vi "sv_Filter Even-Angle Signal for Specific Notch.vi"(0 "even-angle signals":cluster{"r0":dbl, "dr":dbl, "Y":dbl[]}[](array[cluster]), 2 "reset?":bool, 7 "even-angle position info":T1, 9 "notch harmonic":dbl=1.0 format="%0.2f", 11 "error in (no error)":errorcluster, 12 "bandwidth [order]":dbl=1.0 format="%0.2f", 13 "zero delay? (F)":bool) -> (4 "even-angle signals out":cluster{"r0":dbl, "dr":dbl, "Y":dbl[]}[](array[cluster]), 8 "even-angle position info out":T1, 10 "delay [samples]":i32, 15 "error out":errorcluster)   [LabVIEW 2017, in "SoundVib_ContSweptSine.lvlib"]
uses:
  <vilib>/addons/Sound and Vibration/svt_Continuous Swept Sine/SoundVib_ContSweptSine.lvlib
  <vilib>/addons/Sound and Vibration/Order Analysis/Misc/OAT Position Info.ctl
  <vilib>/Analysis/3filter.llb/FIR Filter with I.C. (DBL).vi
  <vilib>/Analysis/NI_AALBase.lvlib
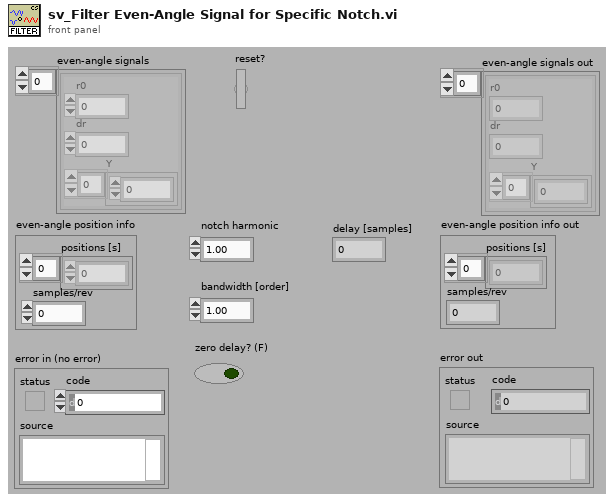
[diagram p1: front panel]
types:
  T1 = typedef "OAT Position Info.ctl" = cluster{"positions [s]":dbl[], "samples/rev":dbl}
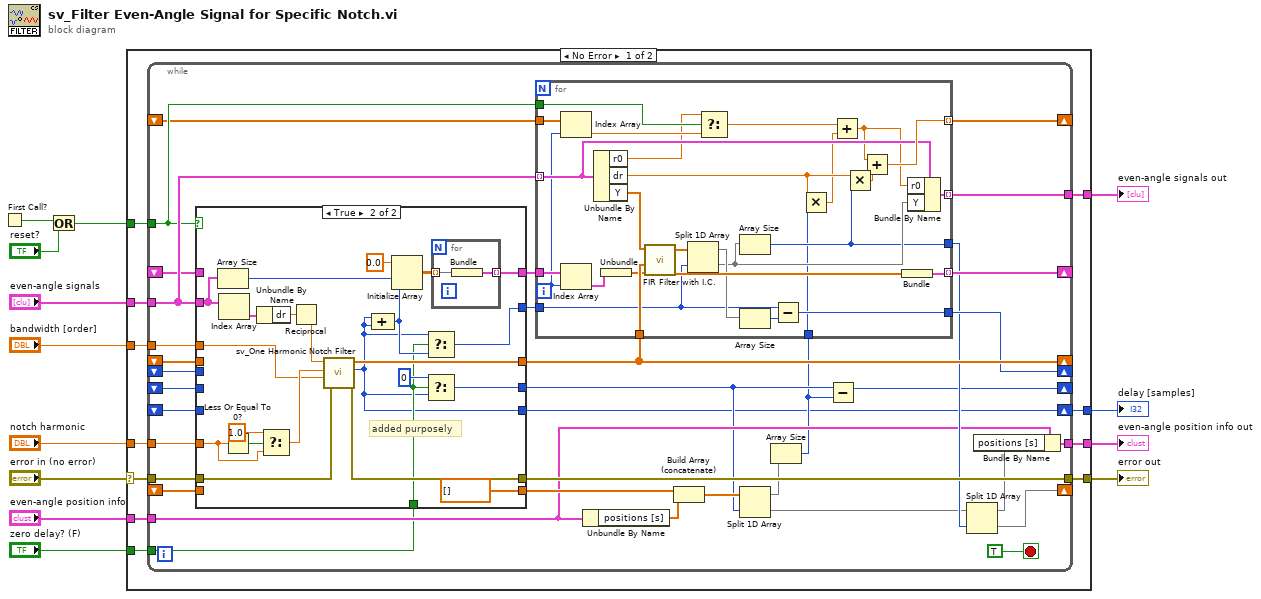
[diagram p0: block diagram]
diagram:
  n1 = First Call?() -> (First Call?: T/F=w13:bool)
  n2 = Or(x=w13, y="reset?") -> (x .or. y?=w11:bool)
  n3 = case shown="No Error" "error in (no error)" {
    selector: "error in (no error)" -> [w20 w123]
    tunnel: w11 -> [w24 _]
    tunnel: "even-angle signals" -> [w23 w122]
    tunnel: "notch harmonic" -> [w22 _]
    tunnel: [w21 w122] -> w8
    tunnel: [w19 w123] -> w6
    tunnel: "even-angle position info" -> [w18 w121]
    tunnel: [w17 w121] -> w4
    tunnel: "zero delay? (F)" -> [w16 _]
    tunnel: [w15 _] -> w2
    tunnel: "bandwidth [order]" -> [w14 _]
    frame No Error {
      n4 = while {
        tunnel: w24 -> [w52]
        tunnel: w23 -> [w55]
        tunnel: w22 -> [w59]
        shift-right: [w54] -> _
        shift-left: _ -> [w58]
        shift-right: [w53] -> _
        shift-left: _ -> [w48]
        shift-right: [w56] -> _
        shift-left: _ -> [w47]
        shift-right: [w51] -> _
        shift-left: _ -> [w50]
        tunnel: [w49] -> w21
        tunnel: w20 -> [w46]
        tunnel: [w45] -> w19
        tunnel: w18 -> [w37]
        shift-right: [w42] -> _
        shift-left: _ -> [w41]
        tunnel: [w36] -> w17
        shift-right: [w32] -> _
        shift-left: _ -> [w31]
        tunnel: w16 -> [w30]
        shift-right: [w25] -> w15
        shift-left: _ -> [w27]
        tunnel: w14 -> [w26]
        stop <- TRUE stop-if-true
        n5 = case shown="True" w52 {
          tunnel: w55 -> [_ w114]
          tunnel: w59 -> [_ w107]
          tunnel: [w95 w116] -> w54
          tunnel: w58 -> [w95 _]
          tunnel: [w94 w111] -> w57
          tunnel: w48 -> [w90 _]
          tunnel: w47 -> [w94 _]
          tunnel: w46 -> [w93 w110]
          tunnel: [w93 w109] -> w45
          tunnel: w41 -> [w92 _]
          tunnel: [w92 dbl[] []] -> w39
          tunnel: [w91 w99] -> w35
          tunnel: w31 -> [w91 _]
          tunnel: w30 -> [_ w100]
          tunnel: [w90 w102] -> w29
          tunnel: w27 -> [w89 _]
          tunnel: w26 -> [_ w97]
          tunnel: [w89 w96] -> w25
          frame False {
          }
          frame True {
            # "added purposely"
            n6 = Array Size(array=w114) -> (size(s)=w113:i32)
            n7 = Index Array(array=w114) -> (element=w118:cluster{"r0":dbl, "dr":dbl, "Y":dbl[]})  [unwired: 1 in]
            n8 = Less Or Equal To 0?(x=w107) -> (x <= 0?=w108:bool)
            n9 = Unbundle By Name(w118) -> ("dr"=w98:dbl)
            n10 = Select(t=1.0, s=w108, f=w107) -> (s? t:f=w105:dbl)
            n11 = Reciprocal(x=w98) -> (1/x=w117:dbl)
            n12 = call <vilib>:"sv_One Harmonic Notch Filter.vi"("error in (no error)"=w110, "bandwidth [order]"=w97, "specific harmonic"=w105, "fs"=w117) -> ("error out"=w109:errorcluster, "delay [samples]"=w96:i32, "FIR filter"=w116:dbl[])  [unwired: 5 in]
            n13 = Compound Arithmetic op=ADD(w96, w96) -> (w103:i32)
            n14 = Initialize Array(0.0 ("element"), w113, w103) -> (w112:dbl[][])
            n15 = Select(t=w96, s=w100, f=w103) -> (s? t:f=w102:i32)
            n16 = Select(t=0, s=w100, f=w96) -> (s? t:f=w99:i32)
            n17 = for {
              tunnel: w112 -> [w120] mode=indexing
              tunnel: [w119] -> w111 mode=indexing
              n18 = Bundle(w120) -> (w119:cluster{dbl[]})  [unwired: 1 in]
            }
          }
        }
        n19 = Unbundle By Name(w37) -> ("positions [s]"=w44:dbl[])
        n20 = Build Array (concatenate)(w39, w44) -> (w40:dbl[])
        n21 = Split 1D Array(array=w40, index=w35) -> (first subarray=w33:dbl[], second subarray=w34:dbl[])
        n22 = Array Size(array=w33) -> (size(s)=w28:i32)
        n23 = for {
          tunnel: w57 -> [w88]
          tunnel: [w74] -> w56 mode=indexing
          tunnel: w55 -> [w79] mode=indexing
          tunnel: w54 -> [w85]
          tunnel: [w83] -> w53
          tunnel: w52 -> [w77]
          tunnel: [w80] -> w51 mode=indexing
          tunnel: w50 -> [w76]
          tunnel: [w75] -> w49 mode=indexing
          tunnel: [w69] -> w43
          tunnel: w29 -> [w68]
          tunnel: w28 -> [w66]
          i -> [w70]
          n24 = Index Array(array=w76, index=w70) -> (element=w72:dbl)
          n25 = Index Array(array=w88, index=w70) -> (element=w71:cluster{"Final X Conditions":dbl[]})
          n26 = Unbundle By Name(w79) -> ("r0"=w63:dbl, "dr"=w65:dbl, "Y"=w86:dbl[])
          n27 = Unbundle(w71) -> ("Final X Conditions"=w73:dbl[])
          n28 = call-poly <vilib>:"FIR Filter with I.C..vi"("Initial X Conditions"=w73, "FIR Coefficients"=w85, "X"=w86) -> ("Final X Conditions"=w87:dbl[], "Filtered X"=w84:dbl[])  [unwired: 5 in, 1 out]
          n29 = Split 1D Array(array=w84, index=w68) -> (first subarray=w82:dbl[], second subarray=w78:dbl[])
          n30 = Select(t=w63, s=w77, f=w72) -> (s? t:f=w62:dbl)
          n31 = Array Size(array=w78) -> (size(s)=w69:i32)
          n32 = Array Size(array=w82) -> (size(s)=w67:i32)
          n33 = Subtract(x=w68, y=w67) -> (x-y=w83:i32)
          n34 = Multiply(x=w65, y=w66) -> (x*y=w64:dbl)
          n35 = Add(x=w62, y=w64) -> (x+y=w61:dbl)
          n36 = Multiply(x=w65, y=w69) -> (x*y=w81:dbl)
          n37 = Add(x=w61, y=w81) -> (x+y=w80:dbl)
          n38 = Bundle("Final X Conditions"=w87) -> (w74:cluster{"Final X Conditions":dbl[]})  [unwired: 1 in]
          n39 = Bundle By Name(cluster=w79, "r0"=w61, "Y"=w78) -> (w75:cluster{"r0":dbl, "dr":dbl, "Y":dbl[]})
        }
        n40 = Subtract(x=w35, y=w28) -> (x-y=w32:i32)
        n41 = Split 1D Array(array=w34, index=w43) -> (first subarray=w38:dbl[], second subarray=w42:dbl[])
        n42 = Bundle By Name(cluster=w37, "positions [s]"=w38) -> (w36:T1)
      }
    }
    frame Error {
    }
  }
  "even-angle signals out" <- w8
  "error out" <- w6
  "even-angle position info out" <- w4
  "delay [samples]" <- w2
